vi "construct send package.vi"(11 "Send command":string) -> (0 "Function Code":string, 1 "Address":string, 3 "Send package":string)   [LabVIEW 2014, in "HPCNC.lvlib"]
uses:
  HPCNC.lvlib
  mosbusCheckSum.dll
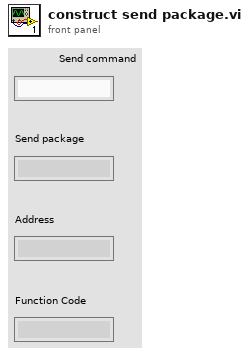
[diagram p1: front panel]
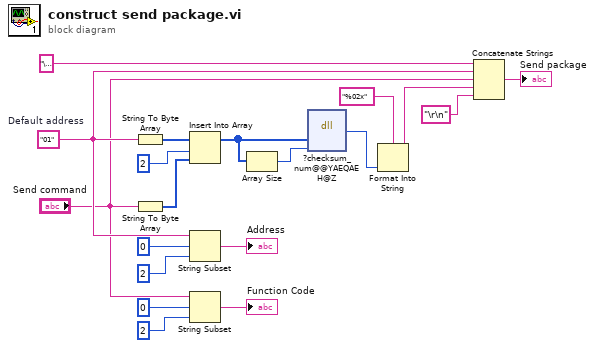
[diagram p0: block diagram]
diagram:
  w13 = "01"  # Default address
  n1 = String To Byte Array(string=w13) -> (unsigned byte array=w19:u8[])
  n2 = String To Byte Array(string="Send command") -> (unsigned byte array=w4:u8[])
  n3 = Insert Into Array(array=w19, index=2, new element=w4) -> (w17:u8[])
  n4 = String Subset(string=w13, offset (0)=0, length (rest)=2 ("length (rest)")) -> (substring=→"Address":string)
  n5 = String Subset(string="Send command", offset (0)=0, length (rest)=2 ("length (rest)")) -> (substring=→"Function Code":string)
  n6 = Array Size(array=w17) -> (size(s)=w16:i32)
  n7 = dll-call lib="D:/Workspace/Giang/Labview/Minigantry With FS/SubVIs/mosbusCheckSum.dll" fn="?checksum_num@@YAEQAEH@Z"("arrayI"=w17, "size"=w16) -> ("return type"=w6:u8)  [unwired: 5 in, 2 out]
  n8 = Format Into String(format string="%02x", w6) -> (resulting string=w2:string)  [unwired: 2 in, 1 out]
  n9 = Concatenate Strings("\u001a", w13, "Send command", w2, "\r\n") -> (→"Send package":string)
